vi "Control Saving.vi"(8 "Error In":errorcluster, 9 "Save":bool) -> (0 "Error Out":errorcluster, 1 "Save status":T1)   [LabVIEW 2015]
panel:
  out "Saving 2":bool
  out "Close File?":bool
  out "Open File?":bool
  out "Saving":bool
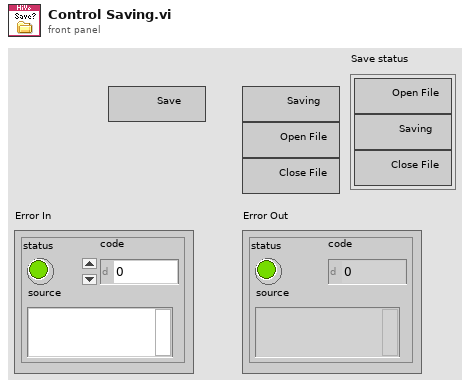
[diagram p1: front panel]
types:
  T1 = cluster{"Saving":bool, "Open File?":bool, "Close File?":bool}
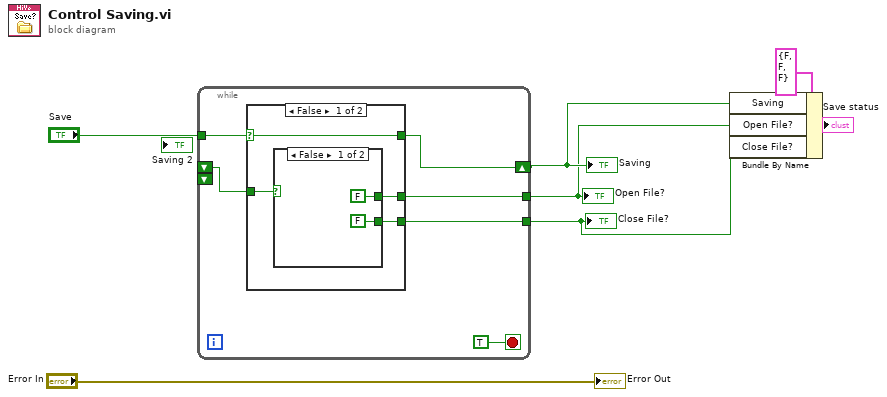
[diagram p0: block diagram]
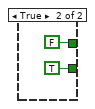
[diagram p2: hidden frame]
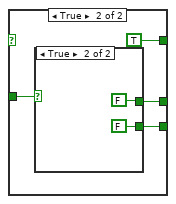
[diagram p3: hidden frame]
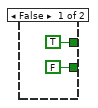
[diagram p4: hidden frame]
diagram:
  n1 = while {
    tunnel: "Save" -> [w12]
    shift-right: [w11] -> w4
    shift-left: _ -> [w10]
    tunnel: [w9] -> w3
    tunnel: [w8] -> w2
    shift-left: _ -> [_]
    stop <- TRUE stop-if-true
    n2 = case shown="False" w12 {
      selector: w12 -> [w14 _]
      tunnel: [w14 TRUE ("Saving 2")] -> w11
      tunnel: w10 -> [w15 w22]
      tunnel: [w17 w24] -> w9
      tunnel: [w16 w23] -> w8
      frame False {
        n3 = case shown="False" w15 {
          tunnel: [FALSE ("Saving 2") FALSE ("Saving 2")] -> w17
          tunnel: [FALSE ("Saving 2") TRUE ("Saving 2")] -> w16
          frame False {
          }
          frame True {
          }
        }
      }
      frame True {
        n4 = case shown="True" w22 {
          tunnel: [TRUE ("Saving 2") FALSE ("Saving 2")] -> w24
          tunnel: [FALSE ("Saving 2") FALSE ("Saving 2")] -> w23
          frame False {
          }
          frame True {
          }
        }
      }
    }
  }
  "Saving" <- w4
  "Open File?" <- w3
  "Close File?" <- w2
  n5 = Bundle By Name(cluster=T1 {"Saving"=FALSE, "Open File?"=FALSE, "Close File?"=FALSE} ("Save status"), "Saving"=w4, "Open File?"=w3, "Close File?"=w2) -> (→"Save status":T1)
  "Error Out" <- "Error In"
